vi "111.vi"() -> ()   [LabVIEW 2017]
panel:
  in  "stop":bool
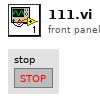
[diagram p1: front panel]
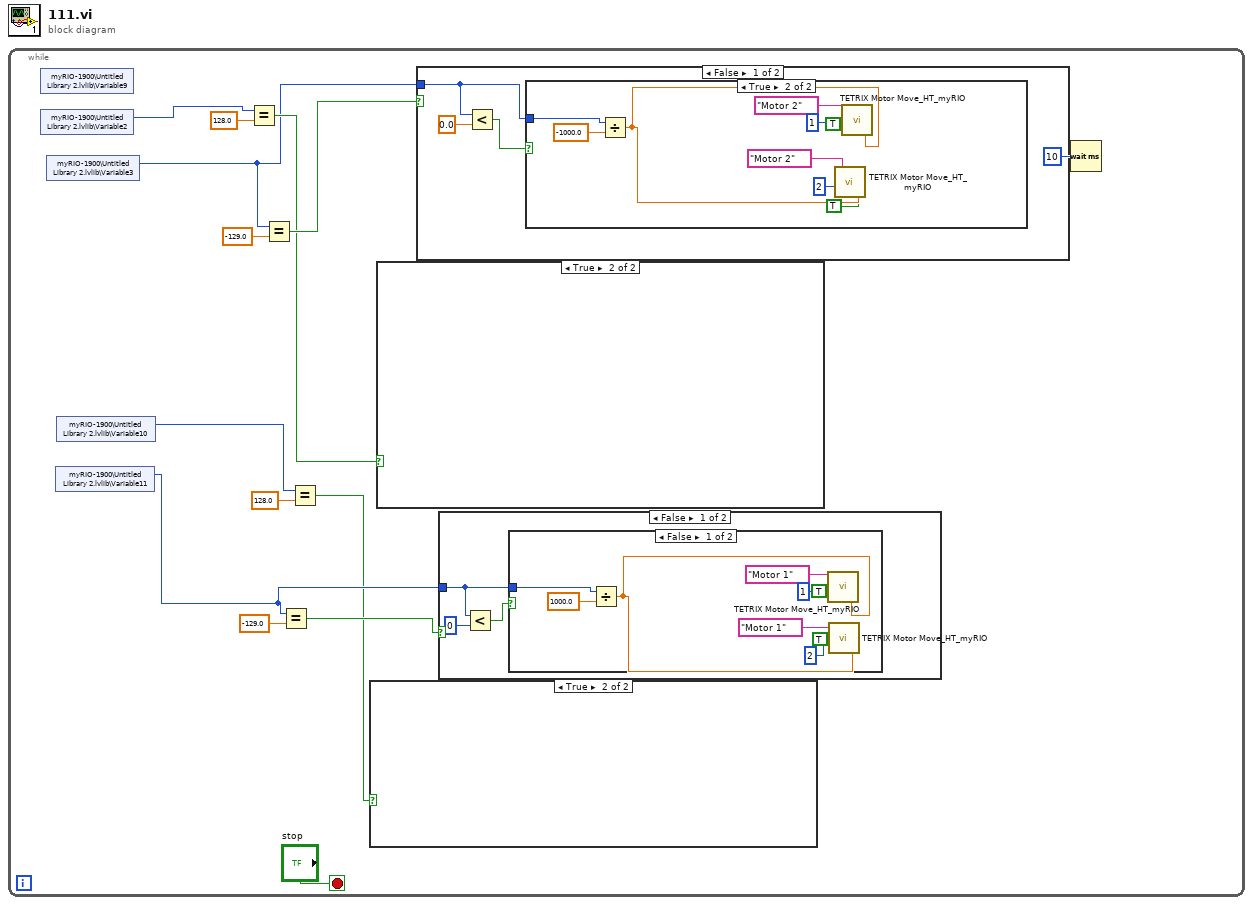
[diagram p0: block diagram]
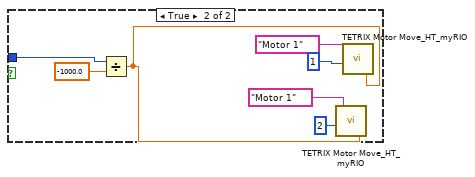
[diagram p3: hidden frame]
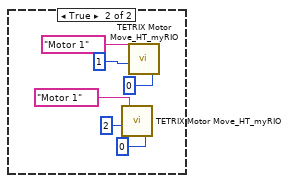
[diagram p4: hidden frame]
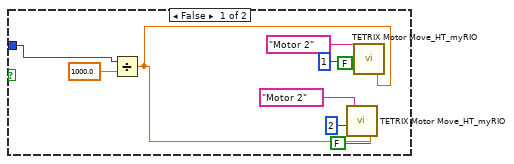
[diagram p6: hidden frame]
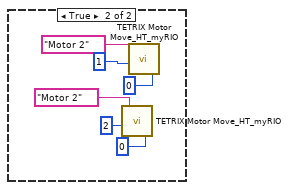
[diagram p7: hidden frame]
diagram:
  n1 = while {
    stop <- "stop" stop-if-true
    n2 = shared-variable "myRIO-1900\\Untitled Library 2.lvlib\\Variable9"() -> ()  [unwired: 1 in, 2 out]
    n3 = shared-variable "myRIO-1900\\Untitled Library 2.lvlib\\Variable2"() -> (w8:i32)  [unwired: 1 in, 1 out]
    n4 = shared-variable "myRIO-1900\\Untitled Library 2.lvlib\\Variable3"() -> (w1:i32)  [unwired: 1 in, 1 out]
    n5 = shared-variable "myRIO-1900\\Untitled Library 2.lvlib\\Variable11"() -> (w7:i32)  [unwired: 1 in, 1 out]
    n6 = shared-variable "myRIO-1900\\Untitled Library 2.lvlib\\Variable10"() -> (w9:i32)  [unwired: 1 in, 1 out]
    n7 = Equal?(x=w8, y=128.0) -> (x = y?=w3:bool)
    n8 = Equal?(x=w1, y=-129.0) -> (x = y?=w4:bool)
    n9 = Equal?(x=w7, y=-129.0) -> (x = y?=w5:bool)
    n10 = Equal?(x=w9, y=128.0) -> (x = y?=w2:bool)
    n11 = case shown="True" w2 {
      frame False {
      }
      frame True {
      }
    }
    n12 = case shown="True" w3 {
      frame False {
      }
      frame True {
      }
    }
    n13 = case shown="False" w4 {
      tunnel: w1 -> [w40 _]
      frame False {
        n14 = Less?(x=w40, y=0.0) -> (x < y?=w42:bool)
        n15 = case shown="True" w42 {
          tunnel: w40 -> [w45 w55]
          frame False {
            n16 = Divide(x=w45, y=1000.0) -> (x/y=w46:dbl)
            n17 = call <vilib>:"TETRIX Motor Move_HT_myRIO.vi"("Power (-100 to 100)\n0 = Stop/Brake\n-128 = Stop/Coast"=w46, "Reverse? : T or F"=FALSE, "Controller Daisy Chain Position: 1 - 4"=u8 2, "Select Channel"="Motor 2") -> ()  [unwired: 3 in, 1 out]
            n18 = call <vilib>:"TETRIX Motor Move_HT_myRIO.vi"("Power (-100 to 100)\n0 = Stop/Brake\n-128 = Stop/Coast"=w46, "Reverse? : T or F"=FALSE, "Controller Daisy Chain Position: 1 - 4"=u8 1, "Select Channel"="Motor 2") -> ()  [unwired: 3 in, 1 out]
          }
          frame True {
            n19 = Divide(x=w55, y=-1000.0) -> (x/y=w54:dbl)
            n20 = call <vilib>:"TETRIX Motor Move_HT_myRIO.vi"("Power (-100 to 100)\n0 = Stop/Brake\n-128 = Stop/Coast"=w54, "Reverse? : T or F"=TRUE, "Controller Daisy Chain Position: 1 - 4"=u8 2, "Select Channel"="Motor 2") -> ()  [unwired: 3 in, 1 out]
            n21 = call <vilib>:"TETRIX Motor Move_HT_myRIO.vi"("Power (-100 to 100)\n0 = Stop/Brake\n-128 = Stop/Coast"=w54, "Reverse? : T or F"=TRUE, "Controller Daisy Chain Position: 1 - 4"=u8 1, "Select Channel"="Motor 2") -> ()  [unwired: 3 in, 1 out]
          }
        }
      }
      frame True {
        n22 = call <vilib>:"TETRIX Motor Move_HT_myRIO.vi"("Power (-100 to 100)\n0 = Stop/Brake\n-128 = Stop/Coast"=i8 0 ("Power (-100 to 100)\n0 = Stop/Brake\n-128 = Stop/Coast"), "Controller Daisy Chain Position: 1 - 4"=u8 2, "Select Channel"="Motor 2") -> ()  [unwired: 4 in, 1 out]
        n23 = call <vilib>:"TETRIX Motor Move_HT_myRIO.vi"("Power (-100 to 100)\n0 = Stop/Brake\n-128 = Stop/Coast"=i8 0 ("Power (-100 to 100)\n0 = Stop/Brake\n-128 = Stop/Coast"), "Controller Daisy Chain Position: 1 - 4"=u8 1, "Select Channel"="Motor 2") -> ()  [unwired: 4 in, 1 out]
      }
    }
    n24 = case shown="False" w5 {
      tunnel: w7 -> [w16 _]
      frame False {
        n25 = Less?(x=w16, y=0) -> (x < y?=w17:bool)
        n26 = case shown="False" w17 {
          tunnel: w16 -> [w20 w27]
          frame False {
            n27 = Divide(x=w20, y=1000.0) -> (x/y=w21:dbl)
            n28 = call <vilib>:"TETRIX Motor Move_HT_myRIO.vi"("Power (-100 to 100)\n0 = Stop/Brake\n-128 = Stop/Coast"=w21, "Reverse? : T or F"=TRUE, "Controller Daisy Chain Position: 1 - 4"=u8 1, "Select Channel"="Motor 1") -> ()  [unwired: 3 in, 1 out]
            n29 = call <vilib>:"TETRIX Motor Move_HT_myRIO.vi"("Power (-100 to 100)\n0 = Stop/Brake\n-128 = Stop/Coast"=w21, "Reverse? : T or F"=TRUE, "Controller Daisy Chain Position: 1 - 4"=u8 2, "Select Channel"="Motor 1") -> ()  [unwired: 3 in, 1 out]
          }
          frame True {
            n30 = Divide(x=w27, y=-1000.0) -> (x/y=w28:dbl)
            n31 = call <vilib>:"TETRIX Motor Move_HT_myRIO.vi"("Power (-100 to 100)\n0 = Stop/Brake\n-128 = Stop/Coast"=w28, "Controller Daisy Chain Position: 1 - 4"=u8 2, "Select Channel"="Motor 1") -> ()  [unwired: 4 in, 1 out]
            n32 = call <vilib>:"TETRIX Motor Move_HT_myRIO.vi"("Power (-100 to 100)\n0 = Stop/Brake\n-128 = Stop/Coast"=w28, "Controller Daisy Chain Position: 1 - 4"=u8 1, "Select Channel"="Motor 1") -> ()  [unwired: 4 in, 1 out]
          }
        }
      }
      frame True {
        n33 = call <vilib>:"TETRIX Motor Move_HT_myRIO.vi"("Power (-100 to 100)\n0 = Stop/Brake\n-128 = Stop/Coast"=i8 0 ("Power (-100 to 100)\n0 = Stop/Brake\n-128 = Stop/Coast"), "Controller Daisy Chain Position: 1 - 4"=u8 2, "Select Channel"="Motor 1") -> ()  [unwired: 4 in, 1 out]
        n34 = call <vilib>:"TETRIX Motor Move_HT_myRIO.vi"("Power (-100 to 100)\n0 = Stop/Brake\n-128 = Stop/Coast"=i8 0 ("Power (-100 to 100)\n0 = Stop/Brake\n-128 = Stop/Coast"), "Controller Daisy Chain Position: 1 - 4"=u8 1, "Select Channel"="Motor 1") -> ()  [unwired: 4 in, 1 out]
      }
    }
    n35 = Wait (ms)(milliseconds to wait=u32 10) -> ()  [unwired: 1 out]
  }
